vi "Set Disable.vi"(8 "error in (no error)":errorcluster, 10 "Disabled":bool, 11 "Element Inhibit in":refnum<class "Element Inhibit.lvclass">) -> (0 "error out":errorcluster, 3 "Element Inhibit out":refnum<class "Element Inhibit.lvclass">)   [LabVIEW 2020, in "VolatusGUI.lvlib" / "Element Inhibit.lvclass"]
uses:
  Element Inhibit.lvclass
  Element Inhibit.lvclass/Element Inhibit.ctl
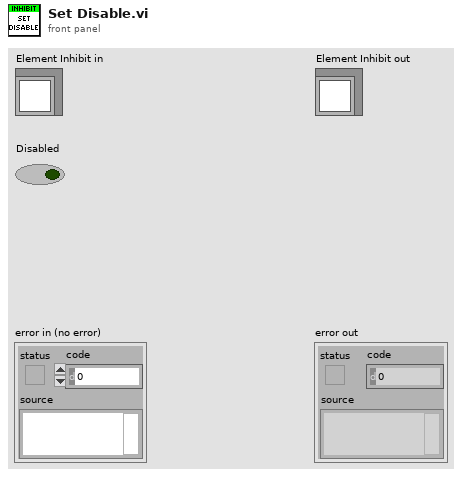
[diagram p1: front panel]
types:
  T1 = enum8{"Enabled", "Disabled", "Disabled and Grayed Out"}
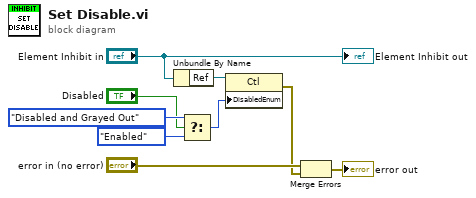
[diagram p0: block diagram]
diagram:
  n1 = Unbundle By Name("Element Inhibit in") -> ("Ref"=w7:refnum<vi>)
  n2 = Select(t=T1."Disabled and Grayed Out" ("Disabled"), s="Disabled", f=T1."Enabled" ("Disabled")) -> (s? t:f=w4:T1)
  n3 = property class="Ctl"(reference=w7, "DisabledEnum"=w4) -> (error out=w1:errorcluster)  [unwired: 1 in, 1 out]
  n4 = Merge Errors("error in (no error)", w1) -> (→"error out":errorcluster)
  "Element Inhibit out" <- "Element Inhibit in"
